vi "ftp tests.vi"() -> ()   [LabVIEW 2015]
uses:
  LabVIEW 3rd Party/LabSSH Library/SFTP Library/Connection Info..cluster.ctl
  LabVIEW 3rd Party/LabSSH Library/SFTP Library/Password..cluster.ctl
  RT VIs/Data Write Control.ctl
  LabVIEW 3rd Party/LabSSH Library/SFTP Library/LabSFTP.lvlib
panel:
  out "target path":string
  out "file write error":errorcluster
  out "path":path
  out "filename":string
  out "isSftpConnected":bool
  in  "Password":T1={"Password"="U-2-id-d"}
  in  "Connection Info.":T2={"Remote"="sec2idd.xray.aps.anl.gov", "Username"="user2idd", "Port (22)"=22}
  out "Connection return":string
  out "Upload return":string
  out "Upload error":errorcluster
  in  "remote path":string="/mnt/xfm0-data2/data/2iddf_Velo"
  in  "dir":string="cRIO-ftp"
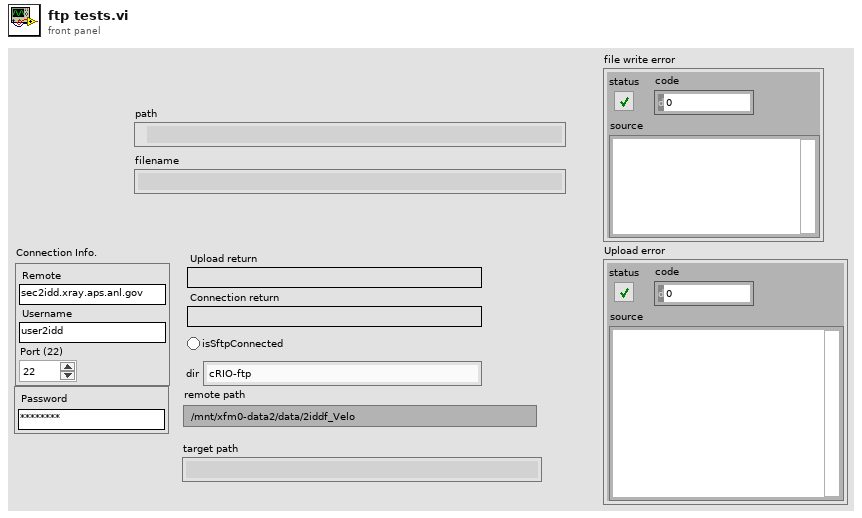
[diagram p1: front panel]
types:
  T1 = typedef "LabSFTP.lvlib/Password..cluster.ctl" = cluster{"Password":string}
  T2 = typedef "LabSFTP.lvlib/Connection Info..cluster.ctl" = cluster{"Remote":string, "Username":string, "Port (22)":i32}
  T3 = typedef "Data Write Control.ctl" = enum16{"Initialize", "Read", "Write", "Close"}
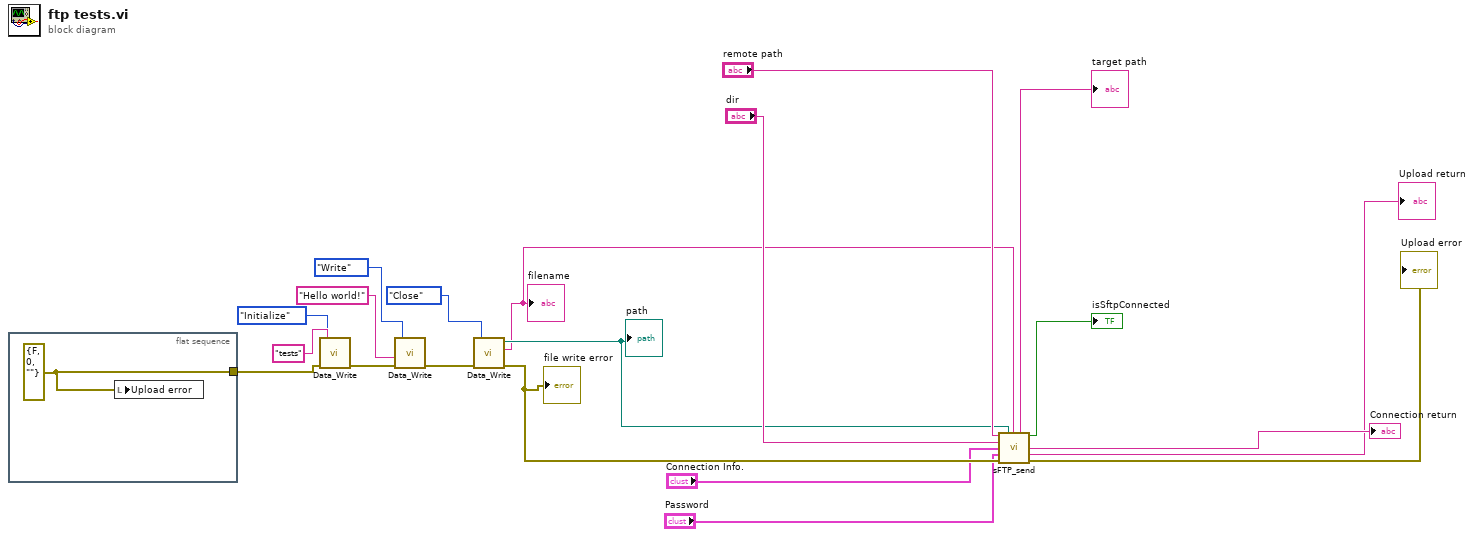
[diagram p0: block diagram]
diagram:
  n1 = flat-sequence {
    tunnel: [w21] -> w12
    frame #0 {
      w21 = errorcluster {"status"=FALSE, "code"=0, "source"=""} ("error initialize")
      n2 = local write "Upload error"(w21) -> ()
    }
  }
  n3 = call "Data_Write.vi"("Command List"=Data_Write_Control."Initialize", "name"="tests", "error initialize"=w12) -> ("error out"=w18:errorcluster)  [unwired: 4 in, 2 out]
  n4 = call "Data_Write.vi"("Command List"=Data_Write_Control."Write", "Data"="Hello world!", "error initialize"=w18) -> ("error out"=w17:errorcluster)  [unwired: 4 in, 2 out]
  n5 = call "Data_Write.vi"("Command List"=Data_Write_Control."Close", "error initialize"=w17) -> ("path"=w7:path, "filename"=w6:string, "error out"=w11:errorcluster)  [unwired: 5 in]
  "filename" <- w6
  "path" <- w7
  "file write error" <- w11
  n6 = call "sFTP_send.vi"("remote path"="remote path", "local path"=w7, "filename"=w6, "dir"="dir", "Connection Info."="Connection Info.", "Password"="Password", "error in (no error)"=w11) -> ("target path"=→"target path":string, "isSftpConnected"=→"isSftpConnected":bool, "Connection return"=→"Connection return":string, "Upload return"=→"Upload return":string, "error out"=→"Upload error":errorcluster)  [unwired: 4 in]
